vi "_ConnectorPaneEditor_Draw_ConnectorPane.vi"(8 "error in (no error)":errorcluster, 11 "ConnectorPaneEditor in":refnum<class "_ConnectorPaneEditor.lvclass">) -> (0 "error out":errorcluster, 1 "CP_Picture":picture, 3 "ConnectorPaneEditor out":refnum<class "_ConnectorPaneEditor.lvclass">, 4 "Pattern":u32)   [LabVIEW 2014, in "_ConnectorPaneEditor.lvclass"]
doc: "Pobiera dane o connector pane z vi o rysuje odpowiednio pokolorowany obraz."
uses:
  _ConnectorPaneEditor.lvclass
  _ConnectorPaneEditor.lvclass/_ConnectorPaneEditor.ctl
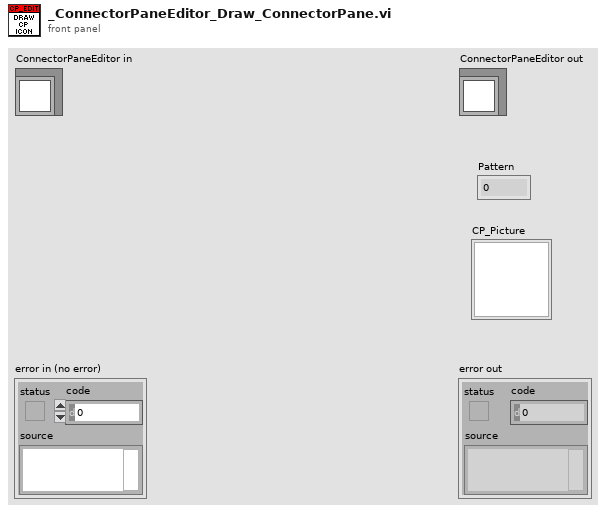
[diagram p1: front panel]
types:
  T1 = cluster{"Width":i16, "Style":enum32{"Solid", "Dash", "Dot", "DashDot", "DashDotDot"}}
  T2 = cluster{"horizontal":enum16{"left", "center", "right"}, "vertical":enum16{"top", "center", "bottom"}}
  T3 = enum16{"User-specified Font", "Application Font", "System Font", "Dialog Font"}
  T4 = cluster{"Font Name:":string, "Size":i16, "Strikeout?":bool, "Italic?":bool, "Underline?":bool, "Outline?":bool, "Shadow?":bool, "Bold?":bool}
  T5 = typedef "LVRectTypeDef.ctl" = cluster{"Left":i16, "Top":i16, "Right":i16, "Bottom":i16}
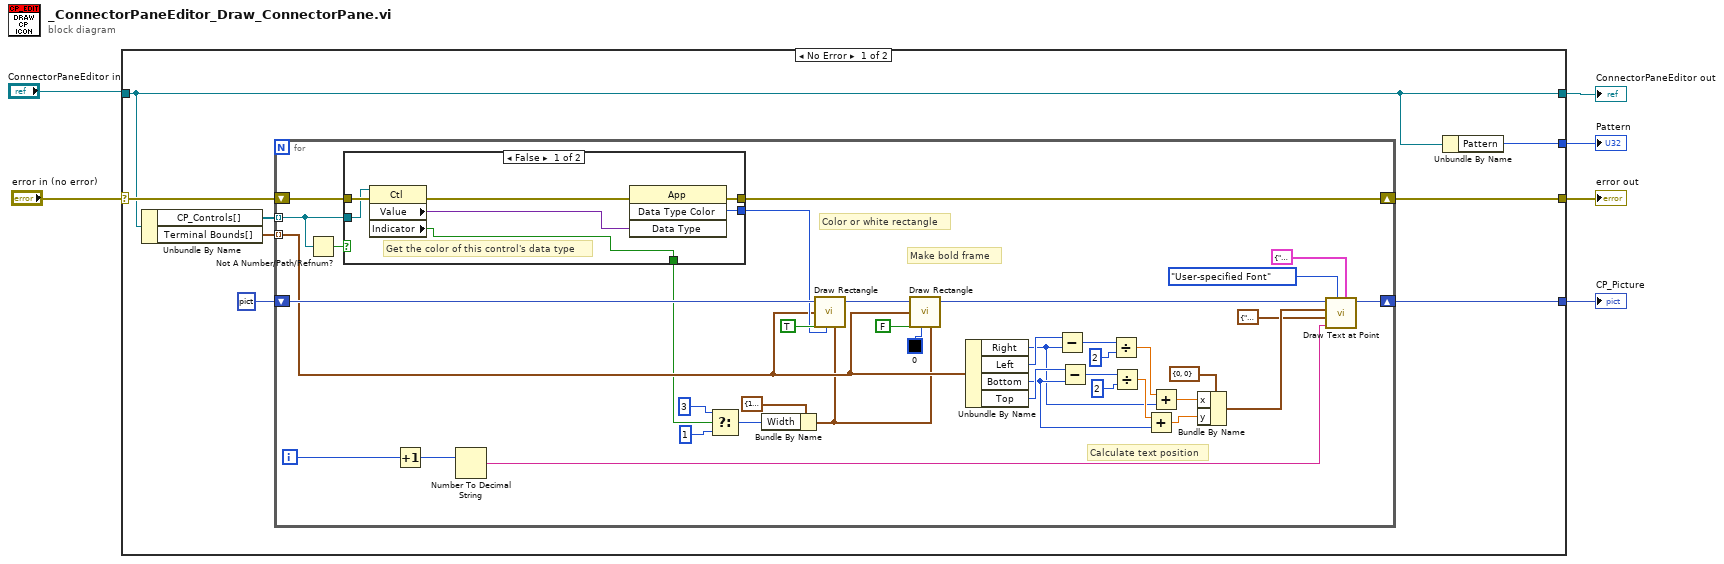
[diagram p0: block diagram]
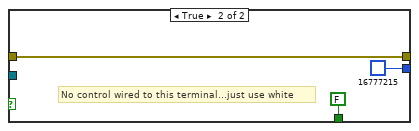
[diagram p2: hidden frame]
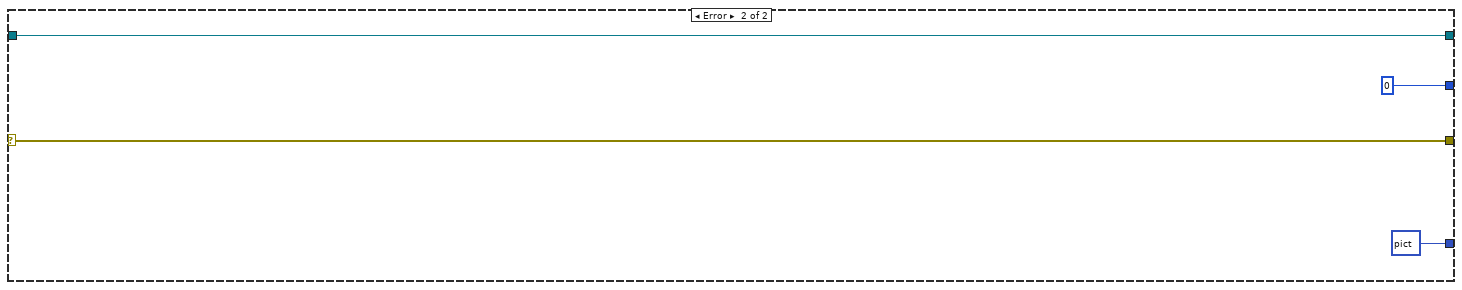
[diagram p3: hidden frame]
diagram:
  n1 = case shown="No Error" "error in (no error)" {
    selector: "error in (no error)" -> [w9 w67]
    tunnel: [w13 w67] -> w3
    tunnel: "ConnectorPaneEditor in" -> [w8 w66]
    tunnel: [w8 w66] -> w4
    tunnel: [w12 picture data[5B] ("empty picture")] -> w2
    tunnel: [w7 u32 0 ("Pattern")] -> w1
    frame No Error {
      n2 = Unbundle By Name(w8) -> ("CP_Controls[]"=w10:refnum<vi>[], "Terminal Bounds[]"=w11:T5[])
      n3 = for {
        tunnel: w11 -> [w34] mode=indexing
        tunnel: w10 -> [w51] mode=indexing
        shift-right: [w50] -> w13
        shift-left: w9 -> [w53]
        shift-right: [w38] -> w12
        shift-left: picture data[5B] ("empty picture") -> [w49]
        i -> [w43]
        # "Calculate text position"
        # "Make bold frame"
        # "Color or white rectangle"
        n4 = Not A Number/Path/Refnum?(number/path/refnum=w51) -> (NaN/Path/Refnum?=w52:bool)
        n5 = case shown="False" w52 {
          tunnel: w53 -> [w60 w63]
          tunnel: w51 -> [w59 _]
          tunnel: [w58 w63] -> w50
          tunnel: [w57 u32 16777215] -> w45
          tunnel: [w56 FALSE ("Indicator")] -> w18
          frame False {
            # "Get the color of this control's data type"
            n6 = property class="Ctl"(reference=w59, error in=w60) -> (error out=w54:errorcluster, "Value"=w55:variant, "Indicator"=w56:bool)  [unwired: 1 out]
            n7 = invoke class="App" method="Data Type Color"(error in=w54, "Data Type"=w55) -> (error out=w58:errorcluster, "Data Type Color"=w57:u32)  [unwired: 2 in, 2 out]
          }
          frame True {
            # "No control wired to this terminal...just use white"
          }
        }
        n8 = Increment(x=w43) -> (x+1=w42:i32)
        n9 = Number To Decimal String(number=w42) -> (decimal integer string=w37:string)  [unwired: 1 in]
        n10 = Select(t=i16 3 ("Width"), s=w18, f=i16 1) -> (s? t:f=w19:i16)
        n11 = Bundle By Name(cluster=T1 {"Width"=1, "Style"=enum."Solid"} ("pen"), "Width"=w19) -> (w15:T1)
        n12 = call <vilib>:"Draw Rectangle.vi"("picture"=w49, "rect"=w34, "fill?(F)"=TRUE, "color(black)"=w45, "pen"=w15) -> ("new picture"=w48:picture)  [unwired: 4 in]
        n13 = call <vilib>:"Draw Rectangle.vi"("picture"=w48, "rect"=w34, "fill?(F)"=FALSE, "color(black)"=u32 0, "pen"=w15) -> ("new picture"=w39:picture)  [unwired: 4 in]
        n14 = Unbundle By Name(w34) -> ("Right"=w21:i16, "Left"=w22:i16, "Bottom"=w23:i16, "Top"=w30:i16)
        n15 = Subtract(x=w22, y=w21) -> (x-y=w29:i16)
        n16 = Subtract(x=w30, y=w23) -> (x-y=w26:i16)
        n17 = Divide(x=w29, y=i16 2) -> (x/y=w27:dbl)
        n18 = Divide(x=w26, y=i16 2) -> (x/y=w24:dbl)
        n19 = Add(x=w24, y=w23) -> (x+y=w32:dbl)
        n20 = Add(x=w27, y=w21) -> (x+y=w33:dbl)
        n21 = Bundle By Name(cluster=cluster{"x":i16, "y":i16} {"x"=0, "y"=0} ("origin"), "x"=w33, "y"=w32) -> (w35:cluster{"x":i16, "y":i16})
        n22 = call <vilib>:"Draw Text at Point.vi"("[user-specified font]"=T4 {"Font Name:"="Arial", "Size"=2, "Strikeout?"=FALSE, "Italic?"=FALSE, "Underline?"=FALSE, "Outline?"=FALSE, "Shadow?"=FALSE, "Bold?"=FALSE}, "desired font(Application)"=T3."User-specified Font", "text"=w37, "alignment(left, top)"=T2 {"horizontal"=enum."center", "vertical"=enum."center"}, "origin"=w35, "picture"=w39) -> ("new picture"=w38:picture)  [unwired: 4 in, 1 out]
      }
      n23 = Unbundle By Name(w8) -> ("Pattern"=w7:u32)
    }
    frame Error {
    }
  }
  "error out" <- w3
  "ConnectorPaneEditor out" <- w4
  "CP_Picture" <- w2
  "Pattern" <- w1
